vi "PicoWritePicoMultiBuffers.vi"(1 "enabled array":i16[](array[numeric]), 2 "Buffer and Transfer Settings":T2={"startIndex"=0, "Samples"=1000000, "Down Sample Ratio"=1, "Down-Sample Mode"=2147483648} {"Down-Sample Mode" items=["RAW none"=2147483648, "None"=0, "Aggregate"=1, "Decimate"=2, "Average"=4]; "Down Sample Ratio" step=1; "Samples" format="%_6p"}, 3 "Variant":string, 5 "Data Pointers":T1, 9 "No of Buffers":i32=1, 11 "error in (no error)":errorcluster, 13 "element value":i16) -> (15 "error out":errorcluster)   [LabVIEW 2010]
doc: "Read data from Picodata buffers for Block and 6000a streaming examples"
uses:
  PicoBuffers.ctl
  Buffer and Transfer Settings.ctl
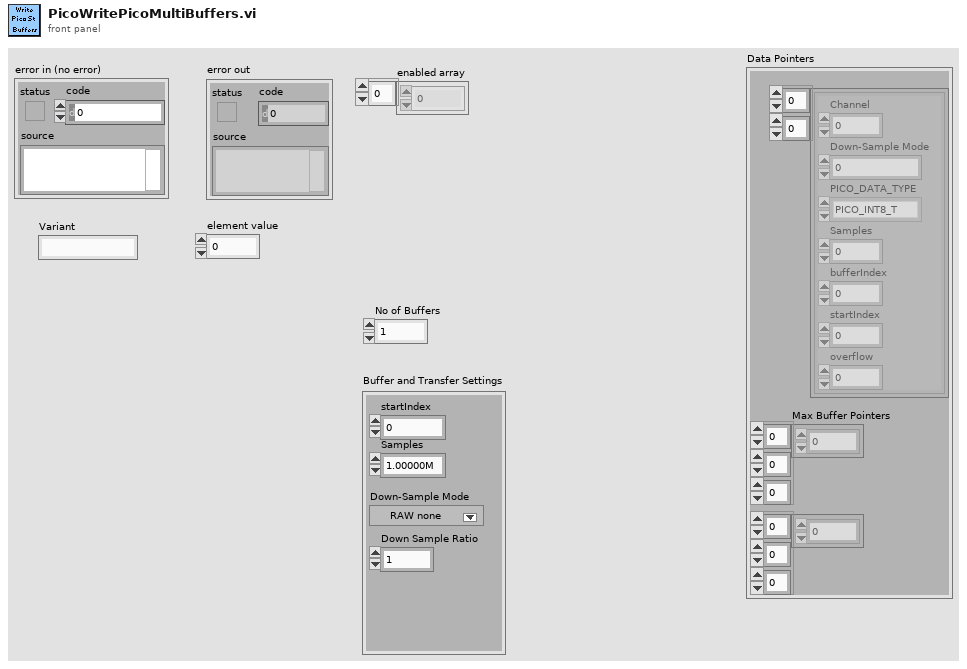
[diagram p1: front panel]
types:
  T1 = typedef "PicoBuffers.ctl" = cluster{"Max Buffer Pointers":u64[][][], "Min Buffer Pointers":u64[][][], "StreamingDataInfo":cluster{"Channel":u32, "Down-Sample Mode":u32, "PICO_DATA_TYPE":enum32{"PICO_INT8_T", "PICO_INT16_T", "PICO_INT32_T", "PICO_UINT32_T", "PICO_INT64_T", ""}, "Samples":i32, "bufferIndex":u64, "startIndex":i32, "overflow":i16}[][]}
  T2 = typedef "Buffer and Transfer Settings.ctl" = cluster{"startIndex":u64, "Samples":u64, "Down Sample Ratio":u64, "Down-Sample Mode":u32}
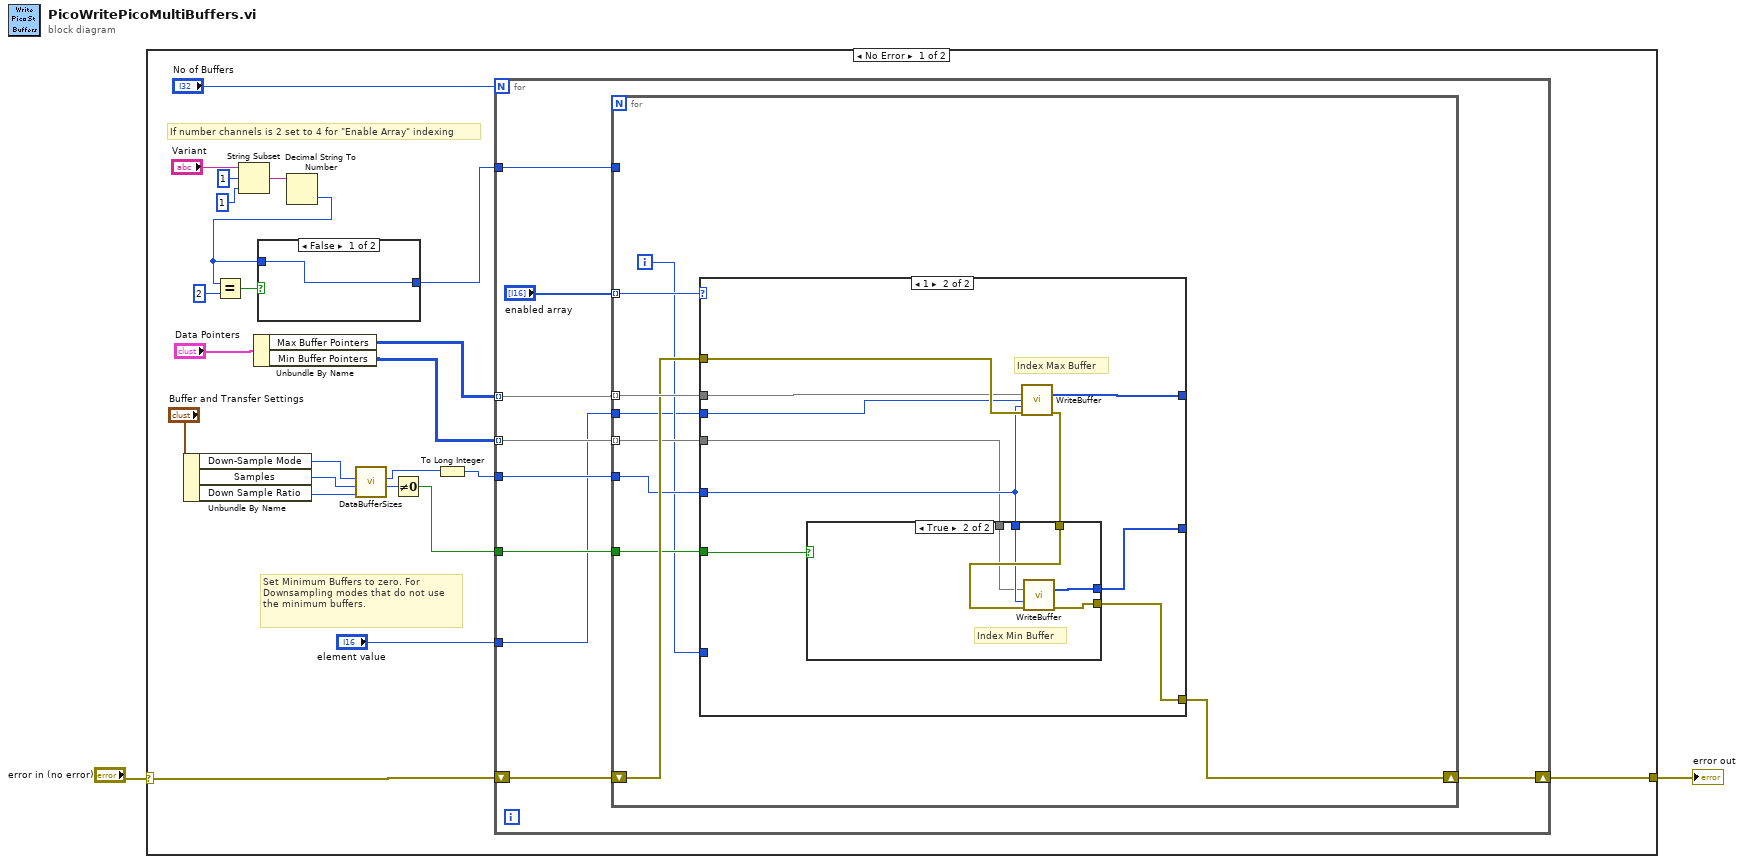
[diagram p0: block diagram]
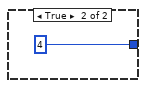
[diagram p2: hidden frame]
diagram:
  n1 = case shown="No Error" "error in (no error)" {
    selector: "error in (no error)" -> [w23 w63]
    tunnel: [w25 w63] -> w1
    frame No Error {
      # "If number channels is 2 set to 4 for \"Enable Array\" indexing"
      # "Set Minimum Buffers to zero. For Downsampling modes that do not use the minimum buffers."
      n2 = Unbundle By Name("Buffer and Transfer Settings") -> ("Down-Sample Mode"=w21:u32, "Samples"=w20:u64, "Down Sample Ratio"=w22:u64)
      n3 = String Subset(string="Variant", offset (0)=1, length (rest)=1 ("length (rest)")) -> (substring=w8:string)
      n4 = Unbundle By Name("Data Pointers") -> ("Max Buffer Pointers"=w13:u64[][][], "Min Buffer Pointers"=w12:u64[][][])
      n5 = Decimal String To Number(string=w8) -> (number=w5:i32)  [unwired: 2 in, 1 out]
      n6 = Equal?(x=w5, y=2 ("Number of channels")) -> (x = y?=w11:bool)
      n7 = case shown="False" w11 {
        tunnel: [w26 4 ("Number of channels")] -> w9
        tunnel: w5 -> [w26 _]
        frame False {
        }
        frame True {
        }
      }
      n8 = call "DataBufferSizes.vi"("Down Sample Ratio"=w22, "Number of Samples"=w20, "Down-Sample Mode"=w21) -> ("min Buffer Size"=w18:i32, "Max Buffer Size"=w15:i32)  [unwired: 7 in]
      n9 = Not Equal To 0?(x=w18) -> (x != 0?=w19:bool)
      n10 = To Long Integer(number=w15) -> (32bit integer=w17:i32)
      n11 = for {
        N: "No of Buffers" -> [_]
        tunnel: w19 -> [w34]
        tunnel: w17 -> [w33]
        shift-right: [w36] -> w25
        shift-left: w23 -> [w35]
        tunnel: w13 -> [w32] mode=indexing
        tunnel: w12 -> [w31] mode=indexing
        tunnel: w9 -> [w30]
        tunnel: "element value" -> [w28]
        n12 = for {
          tunnel: "enabled array" -> [w44] mode=indexing
          tunnel: w32 -> [w45] mode=indexing
          shift-right: [w43] -> w36
          shift-left: w35 -> [w42]
          tunnel: w33 -> [w41]
          tunnel: w34 -> [w40]
          tunnel: w31 -> [w39] mode=indexing
          tunnel: w30 -> [_]
          tunnel: w28 -> [w37]
          i -> [w38]
          n13 = case shown="1" w44 {
            tunnel: w45 -> [_ w49]
            tunnel: w38 -> [_ _]
            tunnel: [_ w56] -> _
            tunnel: [_ w55] -> _
            tunnel: w42 -> [w46 w54]
            tunnel: [w46 w52] -> w43
            tunnel: w41 -> [_ w50]
            tunnel: w40 -> [_ w51]
            tunnel: w39 -> [_ w48]
            tunnel: w37 -> [_ w47]
            frame 0, Default {
            }
            frame 1 {
              # "Index Max Buffer"
              n14 = call "WriteBuffer.vi"("Pointer and BufferSize"=w49, "element"=w47, "Buffer size"=w50, "error in (no error)"=w54) -> ("Pointer and BufferSize Out"=w56:u64[], "error out"=w53:errorcluster)  [unwired: 10 in]
              n15 = case shown="True" w51 {
                tunnel: [_ w62] -> w55
                tunnel: w53 -> [w57 w61]
                tunnel: [w57 w60] -> w52
                tunnel: w50 -> [_ w59]
                tunnel: w48 -> [_ w58]
                frame False {
                }
                frame True {
                  # "Index Min Buffer"
                  n16 = call "WriteBuffer.vi"("Pointer and BufferSize"=w58, "Buffer size"=w59, "error in (no error)"=w61) -> ("Pointer and BufferSize Out"=w62:u64[], "error out"=w60:errorcluster)  [unwired: 11 in]
                }
              }
            }
          }
        }
      }
    }
    frame Error {
    }
  }
  "error out" <- w1
